vi "Add Layer.vi"(8 "error in (no error)":errorcluster, 9 "Behind":bool, 10 "New ShapeRef":refnum<data-value>, 11 "Image in":refnum<class "Image.lvclass">) -> (0 "error out":errorcluster, 3 "Image out":refnum<class "Image.lvclass">)   [LabVIEW 2015, in "LV Image Editor Framework.lvlib" / "Image.lvclass"]
uses:
  Image.lvclass
  Forms/Shape/Shape.lvclass
  Image.lvclass/Image.ctl
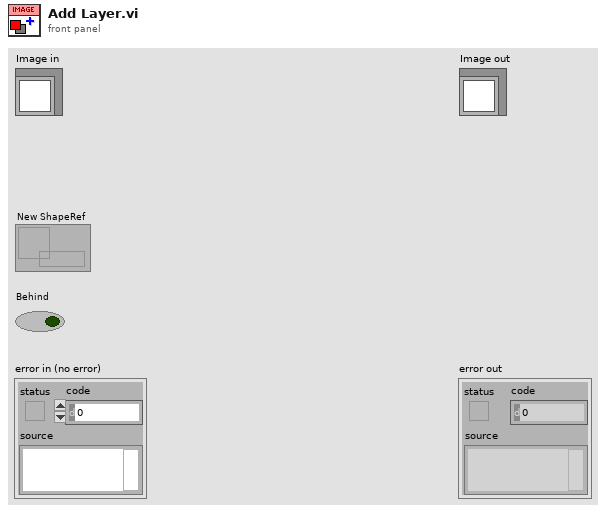
[diagram p1: front panel]
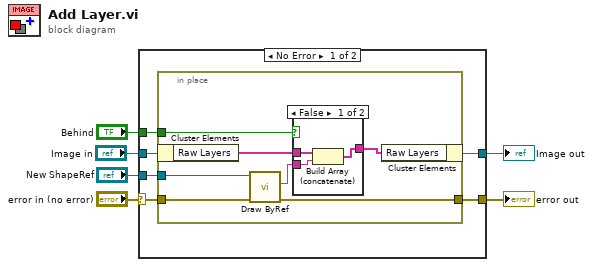
[diagram p0: block diagram]
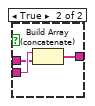
[diagram p2: hidden frame]
diagram:
  n1 = case shown="No Error" "error in (no error)" {
    selector: "error in (no error)" -> [w10 w27]
    tunnel: [w9 w27] -> w5
    tunnel: [w11 w26] -> w3
    tunnel: "Image in" -> [w12 w26]
    tunnel: "New ShapeRef" -> [w8 _]
    tunnel: "Behind" -> [w7 _]
    frame No Error {
      n2 = in-place {
        in-place-border: w10 -> [w17]
        in-place-border: [w16] -> w9
        in-place-border: w8 -> [w14]
        in-place-border: w7 -> [w13]
        n3 = in-place-cluster #1(w12) -> ("Raw Layers"=w19:string[])
        n4 = call "Draw ByRef.vi"("error in (no error)"=w17, "ShapeRef"=w14) -> ("error out"=w16:errorcluster, "Raw Image"=w15:string)  [unwired: 7 in, 1 out]
        n5 = case shown="False" w13 {
          tunnel: w19 -> [w22 w24]
          tunnel: [w21 w23] -> w18
          tunnel: w15 -> [w20 w25]
          frame False {
            n6 = Build Array (concatenate)(w22, w20) -> (w21:string[])
          }
          frame True {
            n7 = Build Array (concatenate)(w25, w24) -> (w23:string[])
          }
        }
        n8 = in-place-cluster #1("Raw Layers"=w18) -> (w11:refnum<class "Image.lvclass">)
      }
    }
    frame Error {
    }
  }
  "error out" <- w5
  "Image out" <- w3
